vi "WriteScanPatternGen.vi"(7 "Error in":errorcluster, 8 "VarParam":string caption="Paramètre de Balayage", 9 "Positions":dbl[](array[numeric]), 10 "Modèle":string) -> (0 "Error out":errorcluster, 2 "SavedOK":bool, 3 "Modèles":string[](array[string]))   [LabVIEW 2019]
doc: "Ce VI sauvegarde les modèles de balayage créer à l'intérieur du fichier de modèles."
uses:
  <vilib>/Utility/config.llb/Write Key (String).vi
  <vilib>/Utility/config.llb/NI_LVConfig.lvlib
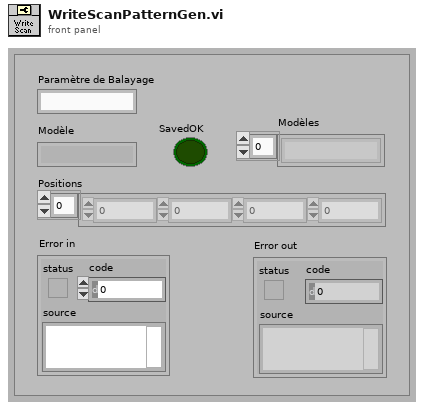
[diagram p1: front panel]
types:
  T1 = typedef "NI_LVConfig.lvlib/Config Data RefNum.ctl" = refnum<k1>
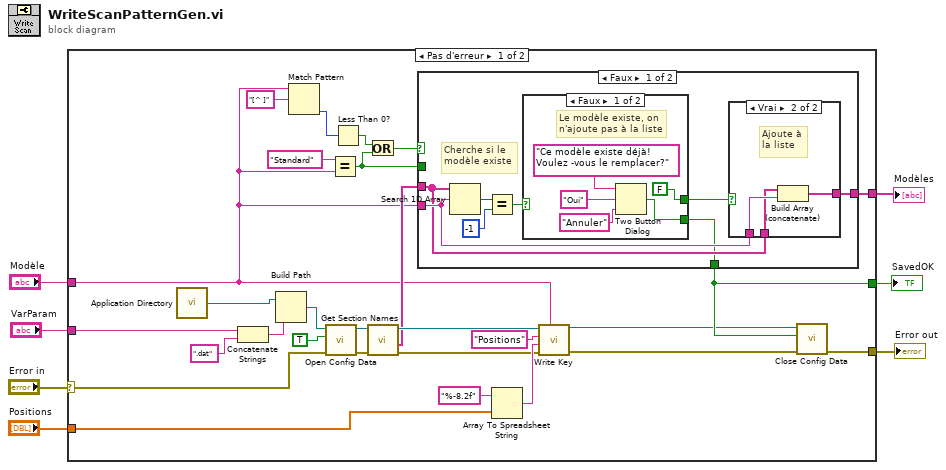
[diagram p0: block diagram]
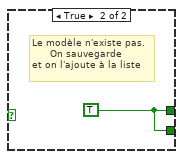
[diagram p3: hidden frame]
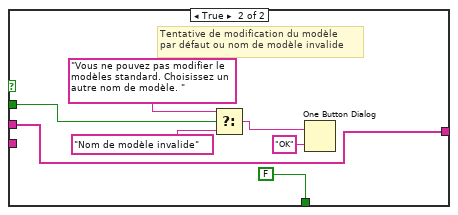
[diagram p4: hidden frame]
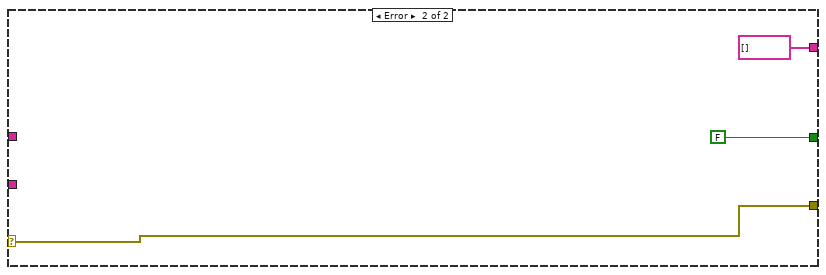
[diagram p5: hidden frame]
diagram:
  n1 = case shown="Pas d'erreur" "Error in" {
    selector: "Error in" -> [w28 w63]
    tunnel: "Modèle" -> [w14 _]
    tunnel: [w32 w63] -> w6
    tunnel: "Positions" -> [w31 _]
    tunnel: [w22 FALSE ("T button?")] -> w3
    tunnel: [w20 string[] [] ("section names")] -> w2
    tunnel: "VarParam" -> [w9 _]
    frame No Error {
      n2 = call <vilib>:"Application Directory.vi"() -> ("Application Directory"=w8:path)
      n3 = Concatenate Strings(w9, ".dat" ("chaîne")) -> (w10:string)
      n4 = Build Path(base path=w8, name or relative path=w10) -> (appended path=w34:path)
      n5 = Match Pattern(string=w14, regular expression="[^ ]") -> (offset past match=w12:i32)  [unwired: 1 in, 3 out]
      n6 = call <vilib>:"Open Config Data.vi"("error in (no error)"=w28, "create file if necessary (T)"=TRUE ("create file if necessary? (T)"), "configuration file path"=w34) -> ("error out"=w27:errorcluster, "refnum"=w24:T1)  [unwired: 6 in, 1 out]
      n7 = Equal?(x="Standard", y=w14) -> (x = y?=w16:bool)
      n8 = Less Than 0?(x=w12) -> (x < 0?=w13:bool)
      n9 = Or(x=w13, y=w16) -> (x .or. y?=w17:bool)
      n10 = call <vilib>:"Get Section Names.vi"("error in (no error)"=w27, "refnum"=w24) -> ("error out"=w26:errorcluster, "section names"=w21:string[], "refnum out"=w25:T1)  [unwired: 7 in]
      n11 = case shown="Faux" w17 {
        tunnel: [w37 FALSE] -> w22
        tunnel: w21 -> [w39 w58]
        tunnel: w14 -> [w40 _]
        tunnel: [w38 w58] -> w20
        tunnel: w16 -> [_ w57]
        frame False {
          # "Cherche si le\nmodèle existe"
          n12 = Search 1D Array(1D array=w39, element=w40) -> (index of element=w43:i32)  [unwired: 1 in]
          n13 = Equal?(x=w43, y=-1) -> (x = y?=w41:bool)
          n14 = case shown="Faux" w41 {
            tunnel: [FALSE w53] -> w36
            tunnel: [w49 w53] -> w37
            frame False {
              # "Le modèle existe, on n'ajoute pas à la liste"
              n15 = Two Button Dialog(message="Ce modèle existe déjà! Voulez -vous le remplacer?", 1:"Annuler" ("F button name (\"Cancel\")"), 2:"Oui" ("T button name (\"OK\")")) -> (T button?=w49:bool)
            }
            frame True {
              w53 = TRUE
              # "Le modèle n'existe pas.\n      On sauvegarde\net on l'ajoute à la liste"
            }
          }
          n16 = case shown="Vrai" w36 {
            tunnel: w40 -> [_ w47]
            tunnel: w39 -> [w44 w46]
            tunnel: [w44 w45] -> w38
            frame False {
            }
            frame True {
              # "Ajoute à\nla liste"
              n17 = Build Array (concatenate)(w46, w47) -> (w45:string[])
            }
          }
        }
        frame True {
          # "Tentative de modification du modèle\npar défaut ou nom de modèle invalide"
          n18 = Select(t="Vous ne pouvez pas modifier le modèles standard. Choisissez un autre nom de modèle. " ("message"), s=w57, f="Nom de modèle invalide" ("message")) -> (s? t:f=w54:string)
          n19 = One Button Dialog(message=w54, button name ("OK")="OK") -> ()  [unwired: 1 out]
        }
      }
      n20 = Array To Spreadsheet String(array=w31, 3:"%-8.2f" ("format string")) -> (spreadsheet string=w29:string)  [unwired: 1 in]
      n21 = call-poly <vilib>:"Write Key.vi"("section"=w14, "error in (no error)"=w26, "value"=w29, "key"="Positions", "refnum"=w25) -> ("error out"=w18:errorcluster, "refnum out"=w19:T1)  [unwired: 4 in, 1 out]
      n22 = call <vilib>:"Close Config Data.vi"("error in (no error)"=w18, "write file if changed (T)"=w22, "refnum"=w19) -> ("error out"=w32:errorcluster)  [unwired: 7 in, 1 out]
    }
    frame Error {
    }
  }
  "Error out" <- w6
  "SavedOK" <- w3
  "Modèles" <- w2
